vi "fake image coordinates.vi"(10 "x triangle?":bool, 11 "scan specification":T1={"x amplitude"=100, "x resolution (pixels)"=28, "x offset fly-forward (iterations)"=50, "x offset fly-back (iterations)"=100, "y resolution (nr. of lines)"=80, "y step size"=30, "iterations per pixel"=5, "number of frames"=80, "y offset (pixels)"=0, "number of y-brake lines  (before y-fly-back)"=0, "number y-brake lines (after y-fly-back)"=40, "number of y-fly-back steps"=0, "lines per z step"=1, "number of z/intensity tuples"=228, "number of repetitions (volumes or planes)"=1000, "z step size derived"=32, "choose the beginning of z scan"=FALSE, "number of frames (settings)"=80, "FPGA trajectory?"=TRUE, "Pockels cell voltage (bits)"=0, "Vy min(bits)"=0, "Vz min(bits)"=0}) -> (1 "zcoords":dbl[](array[numeric]), 2 "ycoords":dbl[](array[numeric]), 3 "xcoords":dbl[](array[numeric]))   [LabVIEW 2010]
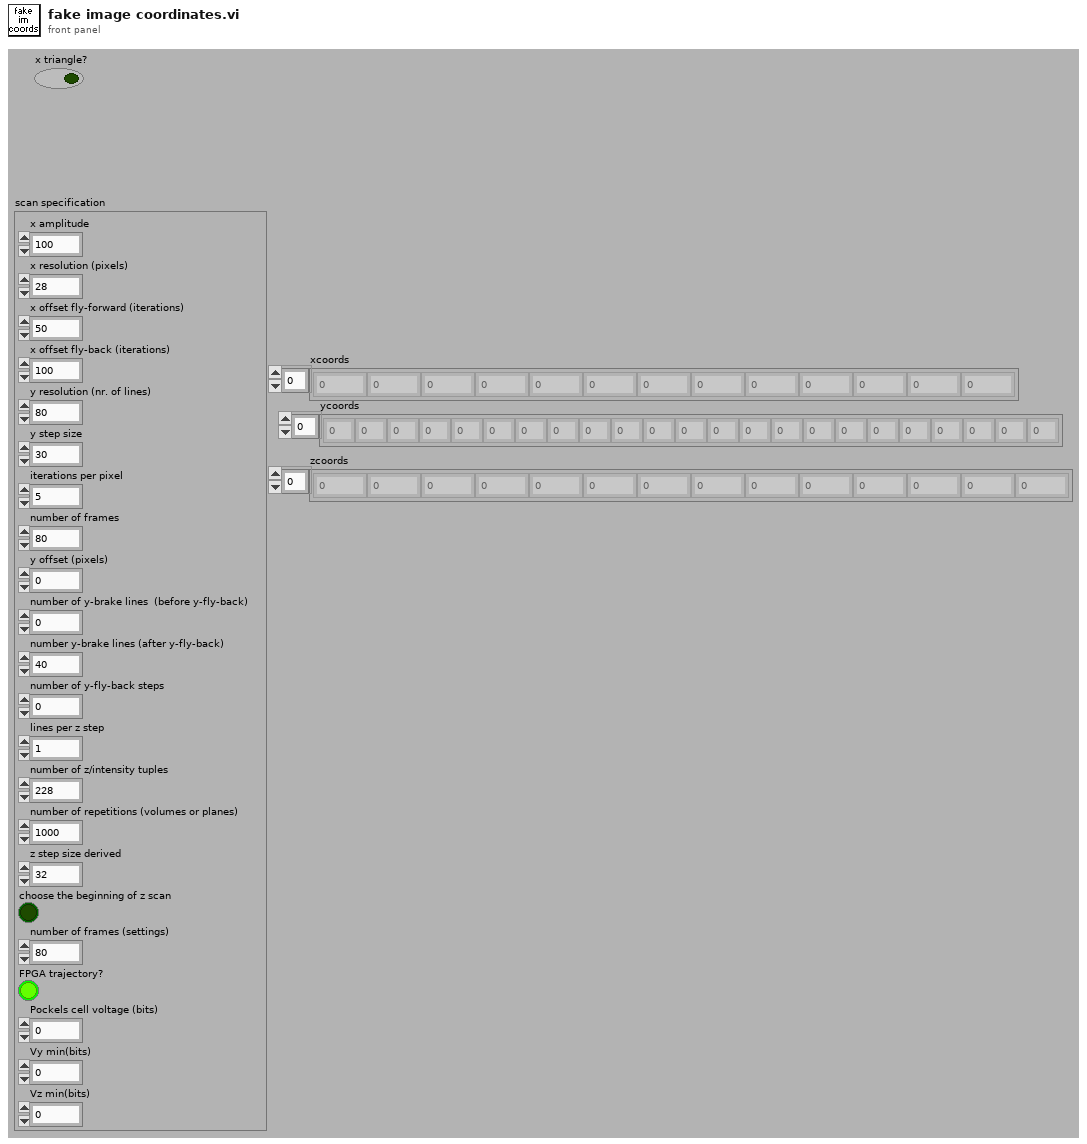
[diagram p1: front panel]
types:
  T1 = cluster{"x amplitude":u16, "x resolution (pixels)":u16, "x offset fly-forward (iterations)":u16, "x offset fly-back (iterations)":u16, "y resolution (nr. of lines)":u16, "y step size":u16, "iterations per pixel":u16, "number of frames":i32, "y offset (pixels)":u16, "number of y-brake lines  (before y-fly-back)":u16, "number y-brake lines (after y-fly-back)":u16, "number of y-fly-back steps":u16, "lines per z step":u16, "number of z/intensity tuples":u16, "number of repetitions (volumes or planes)":i32, "z step size derived":u16, "choose the beginning of z scan":bool, "number of frames (settings)":i32, "FPGA trajectory?":bool, "Pockels cell voltage (bits)":i16, "Vy min(bits)":i16, "Vz min(bits)":i16}
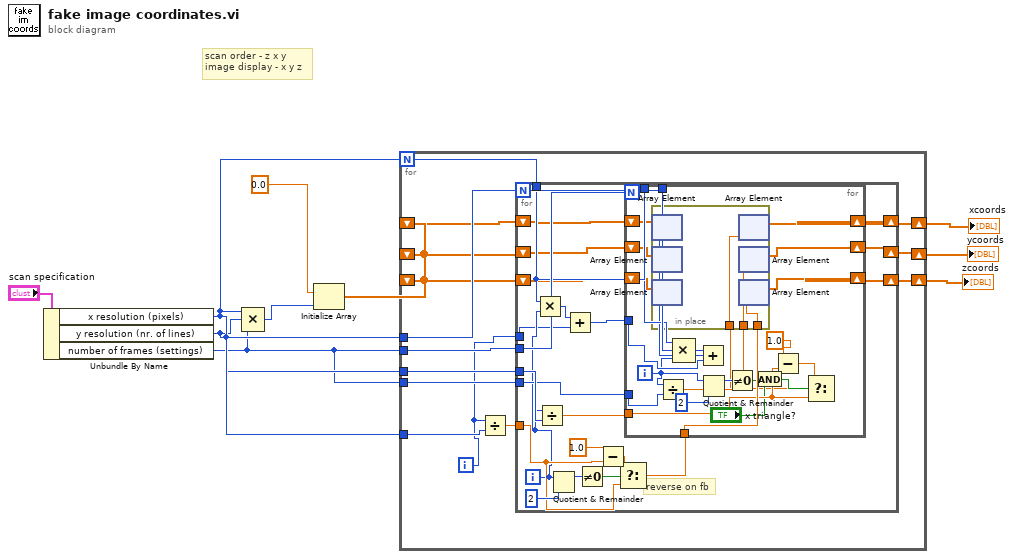
[diagram p0: block diagram]
diagram:
  # "scan order - z x y\nimage display - x y z"
  n1 = Unbundle By Name("scan specification") -> ("x resolution (pixels)"=w7:u16, "y resolution (nr. of lines)"=w6:u16, "number of frames (settings)"=w5:i32)
  n2 = Compound Arithmetic op=MULTIPLY(w7, w6, w5) -> (w8:i32)
  n3 = Initialize Array(0.0, w8) -> (w4:dbl[])
  n4 = for {
    N: w7 -> [w18]
    tunnel: w6 -> [w24]
    tunnel: w5 -> [w23]
    tunnel: w7 -> [w22]
    tunnel: w6 -> [w20]
    tunnel: w5 -> [w19]
    shift-right: [w16] -> w3
    shift-left: w4 -> [w17]
    shift-right: [w14] -> w2
    shift-left: w4 -> [w15]
    shift-right: [w12] -> w1
    shift-left: w4 -> [w13]
    i -> [w11]
    n5 = Divide(x=w11, y=w22) -> (x/y=w21:dbl)
    n6 = for {
      N: w24 -> [w34]
      tunnel: w23 -> [w47]
      tunnel: w21 -> [w41]
      tunnel: w20 -> [w40]
      tunnel: w19 -> [w38]
      tunnel: w11 -> [w35]
      tunnel: w18 -> [w33]
      shift-right: [w30] -> w16
      shift-left: w17 -> [w31]
      shift-right: [w28] -> w14
      shift-left: w15 -> [w29]
      shift-right: [w26] -> w12
      shift-left: w13 -> [w27]
      i -> [w37]
      # "reverse on fb"
      n7 = Multiply(x=w33, y=w37) -> (x*y=w36:i32)
      n8 = Divide(x=w37, y=w40) -> (x/y=w25:dbl)
      n9 = Quotient & Remainder(x=w37, y=2) -> (x-y*floor(x/y)=w45:i32)  [unwired: 1 out]
      n10 = Add(x=w36, y=w35) -> (x+y=w32:i32)
      n11 = Not Equal To 0?(x=w45) -> (x != 0?=w44:bool)
      n12 = Subtract(x=1.0, y=w41) -> (x-y=w42:dbl)
      n13 = Select(t=w42, s=w44, f=w41) -> (s? t:f=w39:dbl)
      n14 = for {
        N: w47 -> [_]
        tunnel: w25 -> [w55]
        tunnel: w39 -> [w61]
        tunnel: w38 -> [w71]
        tunnel: w34 -> [w70]
        tunnel: w33 -> [w69]
        tunnel: w32 -> [w67]
        shift-right: [w60] -> w30
        shift-left: w31 -> [w66]
        shift-right: [w59] -> w28
        shift-left: w29 -> [w65]
        shift-right: [w58] -> w26
        shift-left: w27 -> [w64]
        i -> [w49]
        n15 = Divide(x=w49, y=w71) -> (x/y=w62:dbl)
        n16 = Compound Arithmetic op=MULTIPLY(w69, w70, w49) -> (w68:i32)
        n17 = Add(x=w68, y=w67) -> (x+y=w63:i32)
        n18 = Quotient & Remainder(x=w49, y=2) -> (x-y*floor(x/y)=w50:i32)  [unwired: 1 out]
        n19 = Not Equal To 0?(x=w50) -> (x != 0?=w53:bool)
        n20 = And(x="x triangle?", y=w53) -> (x .and. y?=w51:bool)
        n21 = Subtract(x=1.0, y=w55) -> (x-y=w56:dbl)
        n22 = Select(t=w56, s=w51, f=w55) -> (s? t:f=w48:dbl)
        n23 = in-place {
          in-place-border: w62 -> [w74]
          in-place-border: w61 -> [w73]
          in-place-border: w48 -> [w72]
          n24 = in-place-array #1(w66, w63) -> ()  [unwired: 1 out]
          n25 = in-place-array #2(w65, w63) -> ()  [unwired: 1 out]
          n26 = in-place-array #3(w64, w63) -> ()  [unwired: 1 out]
          n27 = in-place-array #1(w72) -> (w60:dbl[])  [unwired: 1 out]
          n28 = in-place-array #2(w74) -> (w59:dbl[])  [unwired: 1 out]
          n29 = in-place-array #3(w73) -> (w58:dbl[])  [unwired: 1 out]
        }
      }
    }
  }
  "xcoords" <- w3
  "ycoords" <- w2
  "zcoords" <- w1
